vi "Initialise.vi"(8 "error in (no error)":errorcluster, 11 "Index":i32) -> (0 "error out":errorcluster, 3 "Star out":refnum<class "Star.lvclass">)   [LabVIEW 2018, in "Star.lvclass"]
uses:
  Star.lvclass
  C:/dev/PGS/LabMelee v2/Source/Application Specific/Element/Element.lvclass
  Star.lvclass/Star.ctl
  Element/Element.lvclass/Element.ctl
  <vilib>/Utility/file.llb/Application Directory.vi
  Element/Element.lvclass
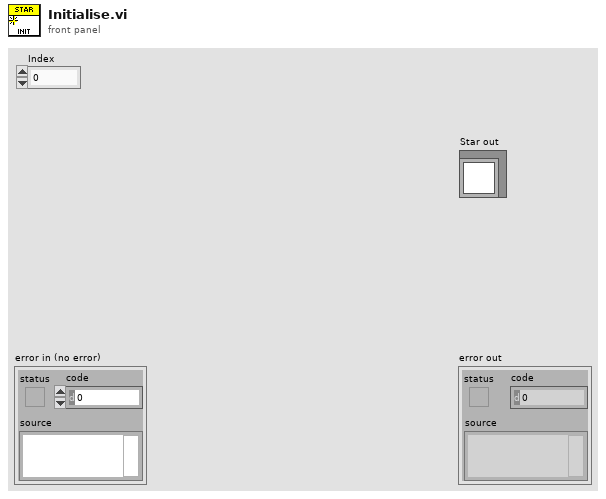
[diagram p1: front panel]
types:
  T1 = typedef "SDL2 Utility.lvlib/Point (I32).ctl" = cluster{"x":i32, "y":i32}
  T2 = typedef "Constants.ctl" = cluster{"Colours":cluster{"OK":u32, "Warning":u32, "Error":u32, "Red":u32, "Green":u32, "Blue":u32, "Yellow":u32}, "System":cluster{"Target Frames Second":dbl, "World Size":T1, "Window Size":T1, "Viewport Size":T1, "Sidebar Scaling":sgl, "Sidebar Width":i32, "SC2 Frame Rate [Seconds/Frame]":sgl}, "Game":cluster{"Maximum Asteroids":i32, "Max Energy":i32, "Max Crew":i32, "Maximum Stars":i32}}
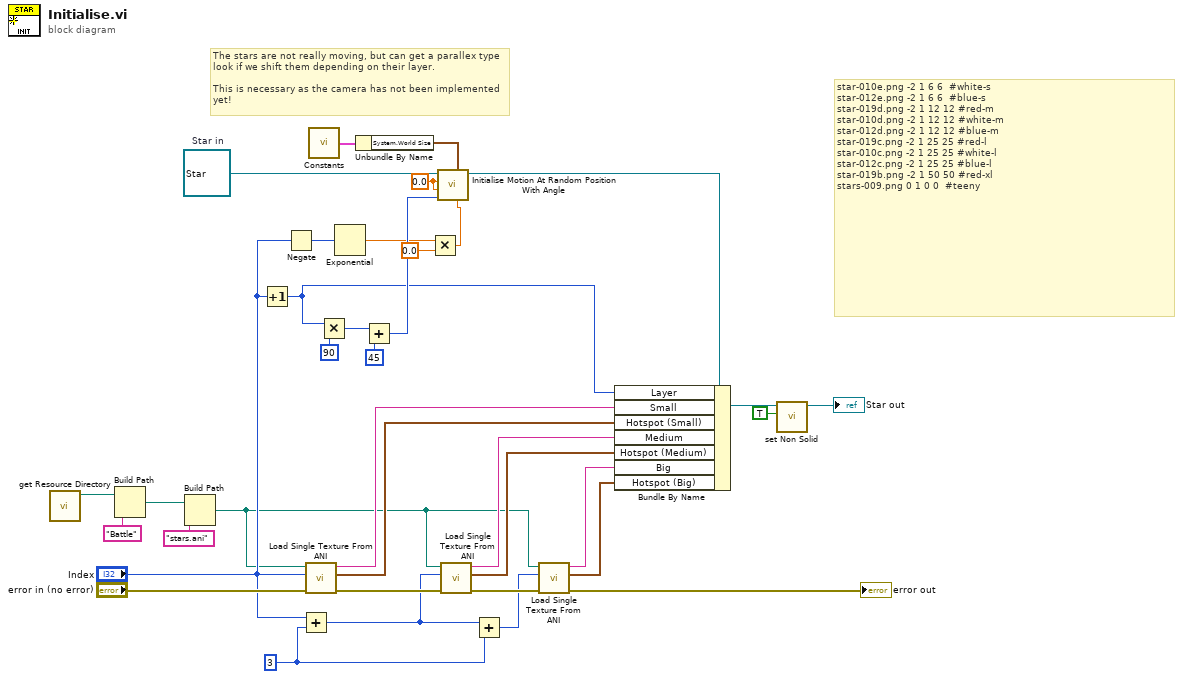
[diagram p0: block diagram]
diagram:
  w3 = 3 ("x")
  w25 = sgl 0.0 ("Turn Rate [deg/s]")
  w35 = refnum<class "Star.lvclass"> refnum  # Star in
  # "star-010e.png -2 1 6 6\t\t#white-s\nstar-012e.png -2 1 6 6\t\t#blue-s\nstar-019d.png -2 1 12 12\t#red-m\nstar-010d.png -2 1 12 12\t#white-m\nstar-012d.png -2 1 12 12\t#blue-m\nstar-019c.png -2 1 25 25\t#red-l\nstar-010c.png -2 1 25 25\t#white-l\nstar-012c.png -2 1 25 25\t#blue-l\nstar-019b.png -2 1 50 50\t#red-xl\nstars-009.png 0 1 0 0\t\t#teeny"
  # "The stars are not really moving, but can get a parallex type look if we shift them depending on their layer.\n\nThis is necessary as the camera has not been implemented yet!"
  n1 = call "get Resource Directory.vi"() -> ("Resource Directory"=w36:path)  [unwired: 11 in]
  n2 = Build Path(base path=w36, name or relative path="Battle") -> (appended path=w31:path)
  n3 = Build Path(base path=w31, name or relative path="stars.ani" ("format string")) -> (appended path=w1:path)
  n4 = Increment(x="Index") -> (x+1=w6:i32)
  n5 = Negate(x="Index") -> (-x=w24:i32)
  n6 = Add(x="Index", y=w3) -> (x+y=w4:i32)
  n7 = call "Load Single Texture From ANI.vi"("error in (no error)"="error in (no error)", "Index"="Index", "Star ANI File"=w1) -> ("error out"=w13:errorcluster, "Hotspot"=w27:T1, "Name In Cache"=w28:string)  [unwired: 6 in]
  n8 = call "Constants.vi"() -> ("Constants"=w32:T2)
  n9 = Multiply(x=w6, y=90) -> (x*y=w22:i32)
  n10 = Exponential(1:w24) -> (0:w19:dbl)
  n11 = Unbundle By Name(w32) -> ("System.World Size"=w30:T1)
  n12 = Add(x=w22, y=45) -> (x+y=w20:i32)
  n13 = Multiply(x=w19, y=0.0) -> (x*y=w17:dbl)
  n14 = call "Initialise Motion At Random Position With Angle.vi"("Initial Velocity [m/s]"=w17, "Field Size"=w30, "Inital Heading [deg]"=w20, "Acceleration [m/s/s]"=w25, "Turn Rate [deg/s]"=w25, "Movable in"=w35) -> ("Movable out"=w34:refnum<class "Star.lvclass">)  [unwired: 5 in]
  n15 = call "Load Single Texture From ANI.vi"("error in (no error)"=w13, "Index"=w4, "Star ANI File"=w1) -> ("error out"=w12:errorcluster, "Hotspot"=w9:T1, "Name In Cache"=w10:string)  [unwired: 6 in]
  n16 = Add(x=w4, y=w3) -> (x+y=w2:i32)
  n17 = call "Load Single Texture From ANI.vi"("error in (no error)"=w12, "Index"=w2, "Star ANI File"=w1) -> ("error out"=→"error out":errorcluster, "Hotspot"=w7:T1, "Name In Cache"=w8:string)  [unwired: 6 in]
  n18 = Bundle By Name(cluster=w34, "Layer"=w6, "Small"=w28, "Hotspot (Small)"=w27, "Medium"=w10, "Hotspot (Medium)"=w9, "Big"=w8, "Hotspot (Big)"=w7) -> (w16:refnum<class "Star.lvclass">)
  n19 = call "set Non Solid.vi"("Non Solid"=TRUE, "Element in"=w16) -> ("Element out"=→"Star out":refnum<class "Star.lvclass">)  [unwired: 9 in]
